vi "Create Camera Image Map.vi"(7 "Action":enum16{"Read", "Write"}(ring), 9 "Image":T1, 11 "key":string) -> (1 "key not found?":bool)   [LabVIEW 2019]
uses:
  <vilib>/vision/Image Controls.llb/IMAQ Image.ctl
panel:
  out "value":T1
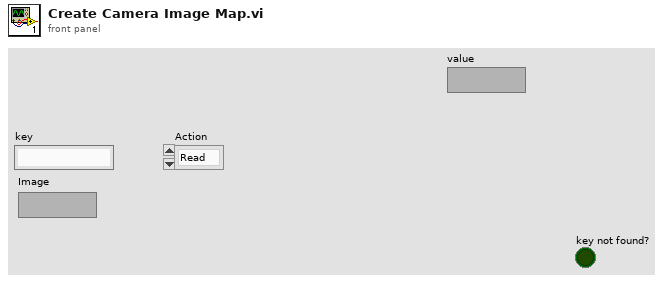
[diagram p1: front panel]
types:
  T1 = typedef "IMAQ Image.ctl" = refnum<image>
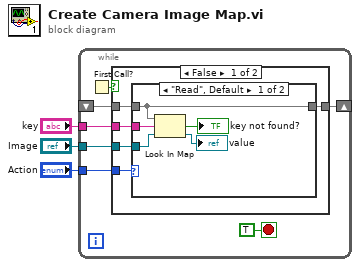
[diagram p0: block diagram]
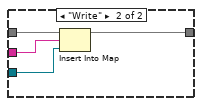
[diagram p2: hidden frame]
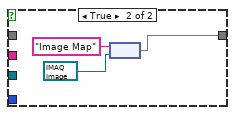
[diagram p3: hidden frame]
diagram:
  n1 = while {
    shift-right: [w7] -> _
    shift-left: _ -> [w8]
    tunnel: "key" -> [w6]
    tunnel: "Action" -> [w5]
    tunnel: "Image" -> [w4]
    stop <- TRUE stop-if-true
    n2 = First Call?() -> (First Call?: T/F=w9:bool)
    n3 = case shown="False" w9 {
      tunnel: w8 -> [w15 _]
      tunnel: [w12 w26] -> w7
      tunnel: w6 -> [w14 _]
      tunnel: w5 -> [w13 _]
      tunnel: w4 -> [w11 _]
      frame False {
        n4 = case shown="\"Read\", Default" w13 {
          tunnel: w15 -> [w18 w24]
          tunnel: w14 -> [w20 w22]
          tunnel: w11 -> [w19 w21]
          tunnel: [w18 w23] -> w12
          frame "Read", Default {
            n5 = Look In Map(map=w18, key=w20, default value=w19) -> (key not found?=→"key not found?":bool, value=→"value":T1)
          }
          frame "Write" {
            n6 = Insert Into Map(map in=w24, key=w22, value=w21) -> (map out=w23:map{string, T1})  [unwired: 2 out]
          }
        }
      }
      frame True {
        n7 = node("Image Map" ("key"), T1 refnum ("s? t:f")) -> (w26:map{string, T1})
      }
    }
  }
